vi "pmbus_write_word_readback.vi"(0 "Device Control session in":refnum<class "Semiconductor Device Control.lvclass">, 5 "reg_u16":T1 {"val" step=1}, 7 "prev success?":bool=TRUE, 11 "error in (no error)":errorcluster) -> (4 "Device Control session out":refnum<class "Semiconductor Device Control.lvclass">, 8 "success?":bool, 15 "error out":errorcluster)   [LabVIEW 2021]
uses:
  <instrlib>/Semi Device Control/Semiconductor Device Control.lvclass
  controls/ltm4676a_reg_u16.ctl
  controls/ltm4676a_reg_uids.ctl
  <instrlib>/Semi Device Control/API/Write Register by Name (Device).vi
  <instrlib>/Semi Device Control/API/Read Register by Name (Device).vi
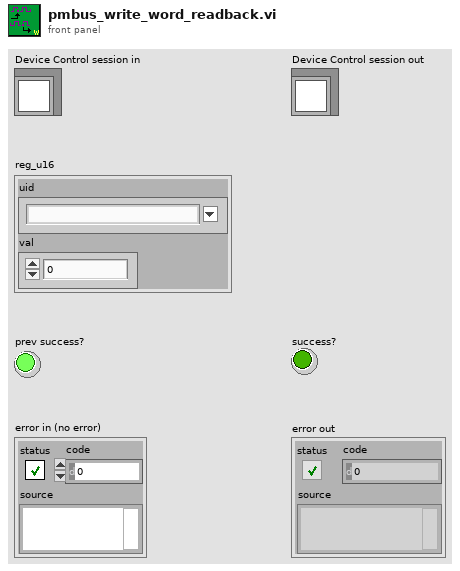
[diagram p1: front panel]
types:
  T1 = typedef "ltm4676a_reg_u16.ctl" = cluster{"uid":T2, "val":u16}
  T2 = typedef "ltm4676a_reg_uids.ctl" = string
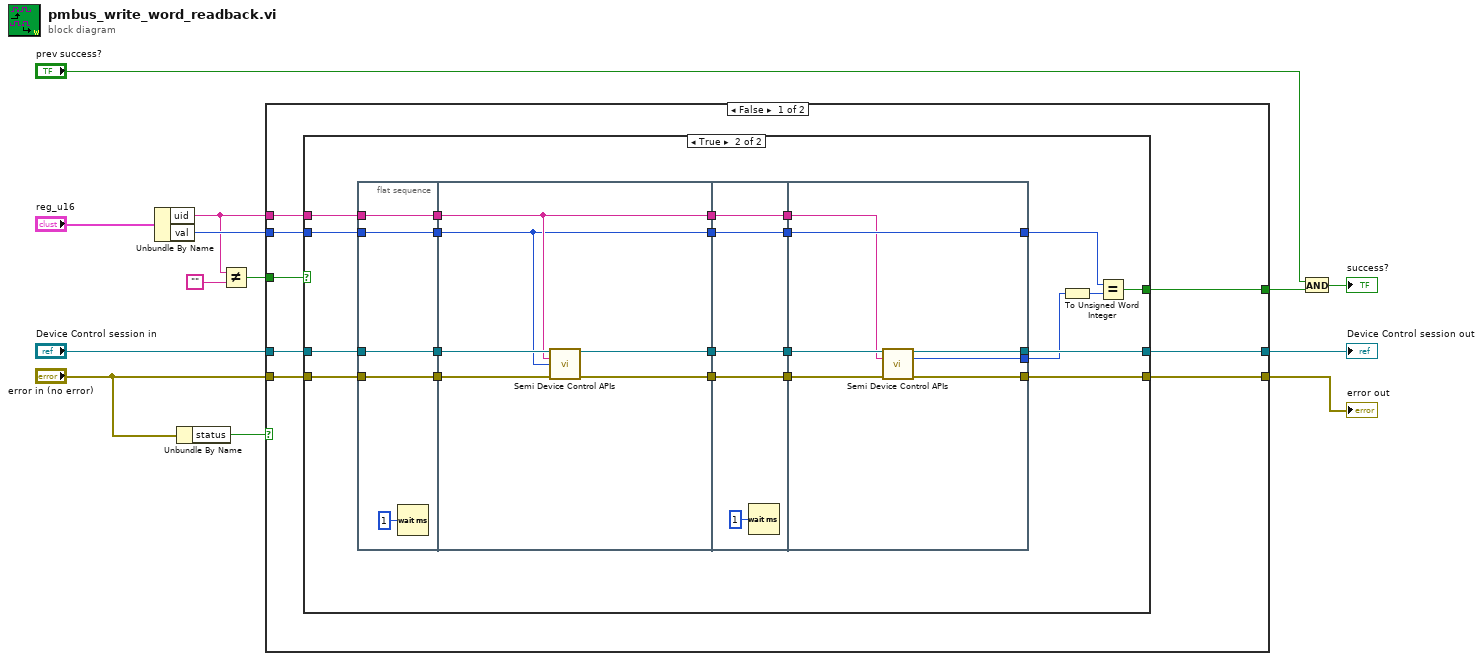
[diagram p0: block diagram]
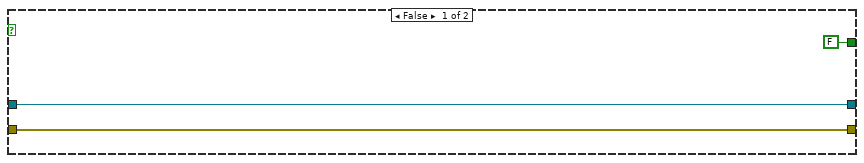
[diagram p2: hidden frame]
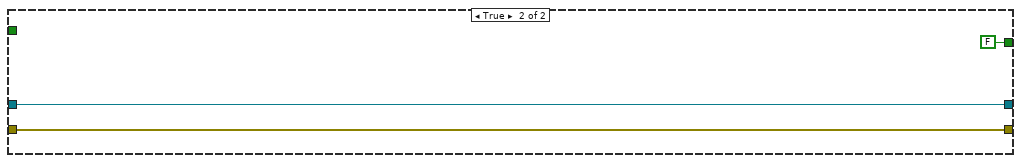
[diagram p3: hidden frame]
diagram:
  n1 = Unbundle By Name("reg_u16") -> ("uid"=w7:T2, "val"=w12:u16)
  n2 = Unbundle By Name("error in (no error)") -> ("status"=w11:bool)
  n3 = Not Equal?(x=w7, y="") -> (x != y?=w6:bool)
  n4 = case shown="False" w11 {
    tunnel: "Device Control session in" -> [w21 w71]
    tunnel: w7 -> [w20 _]
    tunnel: w12 -> [w19 _]
    tunnel: "error in (no error)" -> [w18 w72]
    tunnel: [w17 w71] -> w10
    tunnel: [w16 w72] -> w9
    tunnel: w6 -> [w15 _]
    tunnel: [w14 FALSE] -> w3
    frame False {
      n5 = case shown="True" w15 {
        tunnel: w21 -> [w23 w38]
        tunnel: w20 -> [_ w37]
        tunnel: w19 -> [_ w36]
        tunnel: w18 -> [w22 w35]
        tunnel: [w23 w34] -> w17
        tunnel: [w22 w33] -> w16
        tunnel: [FALSE w25] -> w14
        frame False {
        }
        frame True {
          n6 = flat-sequence {
            tunnel: w36 -> [w48]
            tunnel: w37 -> [w49]
            tunnel: w35 -> [w50]
            tunnel: w38 -> [w51]
            tunnel: [w51] -> w32
            tunnel: [w50] -> w31
            tunnel: [w49] -> w30
            tunnel: [w48] -> w29
            tunnel: [w56] -> w46
            tunnel: [w55] -> w45
            tunnel: [w54] -> w44
            tunnel: [w53] -> w43
            tunnel: w32 -> [w57]
            tunnel: w31 -> [w52]
            tunnel: w30 -> [w54]
            tunnel: w29 -> [w53]
            tunnel: w46 -> [w61]
            tunnel: [w61] -> w42
            tunnel: [w60] -> w41
            tunnel: w45 -> [w60]
            tunnel: w44 -> [w59]
            tunnel: w43 -> [w58]
            tunnel: [w59] -> w40
            tunnel: [w58] -> w39
            tunnel: w42 -> [w69]
            tunnel: w41 -> [w68]
            tunnel: w40 -> [w64]
            tunnel: w39 -> [w65]
            tunnel: [w67] -> w34
            tunnel: [w66] -> w33
            tunnel: [w65] -> w27
            tunnel: [w63] -> w26
            frame #0 {
              n7 = Wait (ms)(milliseconds to wait=u32 1) -> ()  [unwired: 1 out]
            }
            frame #1 {
              n8 = call-poly <instrlib>:"Semi Device Control APIs.vi"("Device Control session in"=w57, "Register UID"=w54, "Register Data"=w53, "error in (no error)"=w52) -> ("Device Control session out"=w56:refnum<class "Semiconductor Device Control.lvclass">, "error out"=w55:errorcluster)  [unwired: 10 in]
            }
            frame #2 {
              n9 = Wait (ms)(milliseconds to wait=u32 1) -> ()  [unwired: 1 out]
            }
            frame #3 {
              n10 = call-poly <instrlib>:"Semi Device Control APIs.vi"("Device Control session in"=w69, "Register UID"=w64, "error in (no error)"=w68) -> ("Device Control session out"=w67:refnum<class "Semiconductor Device Control.lvclass">, "Register Data"=w63:u64, "error out"=w66:errorcluster)  [unwired: 10 in]
            }
          }
          n11 = To Unsigned Word Integer(number=w26) -> (unsigned 16bit integer=w28:u16)
          n12 = Equal?(x=w27, y=w28) -> (x = y?=w25:bool)
        }
      }
    }
    frame True {
    }
  }
  "Device Control session out" <- w10
  "error out" <- w9
  n13 = And(x="prev success?", y=w3) -> (x .and. y?=→"success?":bool)
